vi "Resolve With Error.vi"(8 "error in (no error)":errorcluster, 10 "Error":errorcluster, 11 "Result in":refnum<class "Result.lvclass">) -> (0 "error out":errorcluster)   [LabVIEW 2017, in "Futures.lvlib" / "Result.lvclass"]
doc: "Resolves the result with an error cluster."
uses:
  Result.lvclass
  Result.lvclass/Result.ctl
  Result Data.ctl
  Result Type.ctl
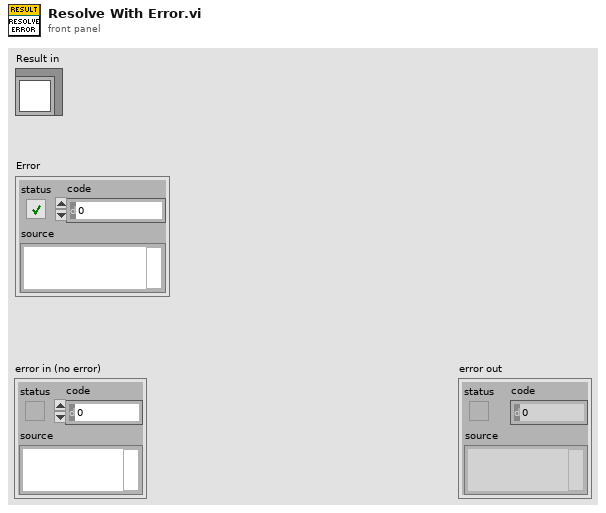
[diagram p1: front panel]
types:
  T1 = typedef "Futures.lvlib/Result.lvclass/Result Type.ctl" = enum16{"Unresolved", "Ok", "Error"}
  T2 = typedef "Futures.lvlib/Result.lvclass/Result Data.ctl" = cluster{"Type":T1, "Value":variant}
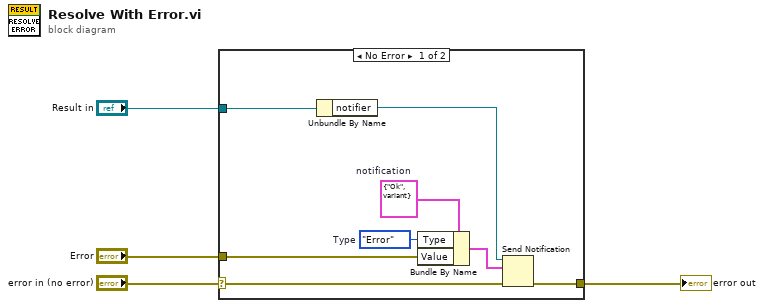
[diagram p0: block diagram]
diagram:
  n1 = case shown="No Error" "error in (no error)" {
    selector: "error in (no error)" -> [w12 w13]
    tunnel: [w11 w13] -> w3
    tunnel: "Result in" -> [w10 _]
    tunnel: "Error" -> [w5 _]
    frame No Error {
      w6 = Result_Type."Error"  # Type
      w8 = T2 {"Type"=enum."Ok", "Value"=variant}  # notification
      n2 = Unbundle By Name(w10) -> ("notifier"=w9:refnum<notifier>)
      n3 = Bundle By Name(cluster=w8, "Type"=w6, "Value"=w5) -> (w7:T2)
      n4 = Send Notification(notification=w7, notifier=w9, error in (no error)=w12) -> (error out=w11:errorcluster)  [unwired: 1 out]
    }
    frame Error {
    }
  }
  "error out" <- w3
